vi "tankdata.vi"(7 "LabVIEW Web Service Request":refnum<class "Web Request.lvclass">) -> ()   [LabVIEW 2019]
uses:
  <vilib>/wsapi/Web Request.lvclass
  Type Defs/JSON_Channel.ctl
  Type Defs/JSON_Pump.ctl
panel:
  # "Use the Web Service Request input terminal to call the VIs on the Web Services palette. Do not remove it from the connector pane unless you don't need access to the palette."
  # "Each additional control wired to the connector pane will be available as an input in the URL. To include an indicator in terminal-mode output (the default setting), it must also be wired to the connector pane."
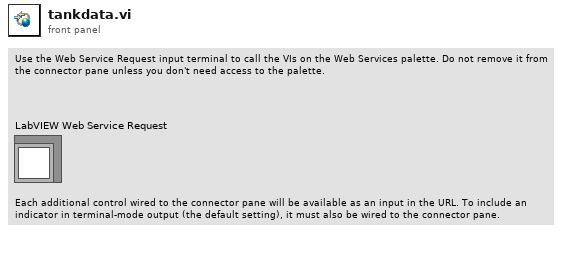
[diagram p1: front panel]
types:
  T1 = typedef "JSON_Tank.ctl" = cluster{"number":u16, "building":string, "room":string, "ipAddress":string, "profileName":string, "caNumber":string, "ctrlType":string, "mode":string, "channels":T2[], "pumps":T3[]}
  T2 = typedef "JSON_Channel.ctl" = cluster{"name":string, "tag":string, "data":string, "type":string, "unit":string}
  T3 = typedef "JSON_Pump.ctl" = cluster{"position":u8, "enabled":bool, "command":string, "channels":T2[], "elapsedTime":string}
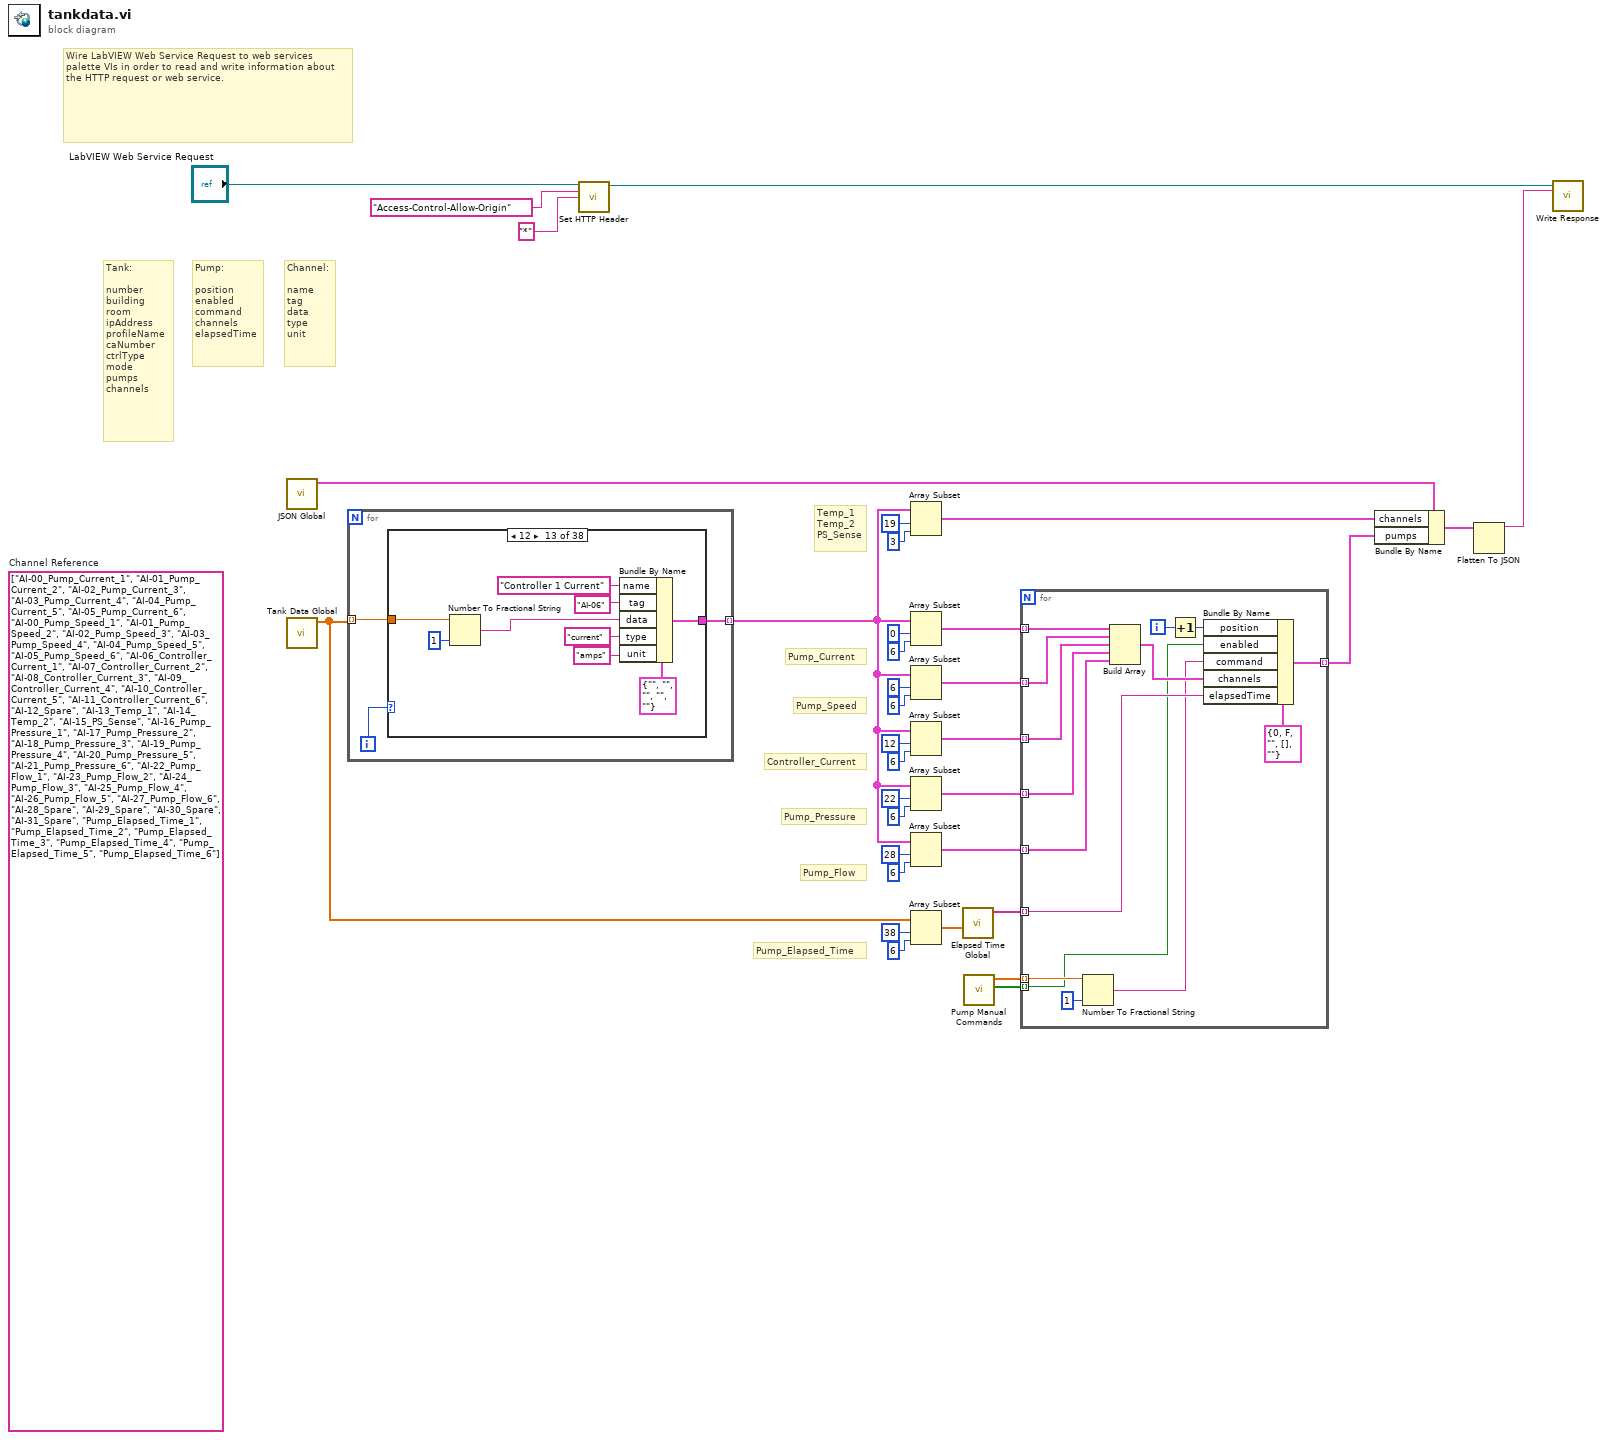
[diagram p0: block diagram]
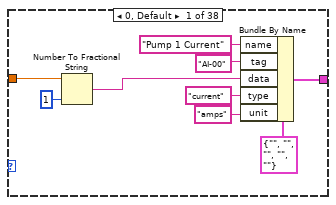
[diagram p2: hidden frame]
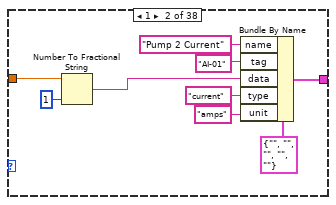
[diagram p3: hidden frame]
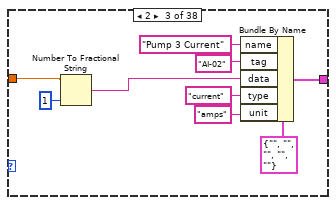
[diagram p4: hidden frame]
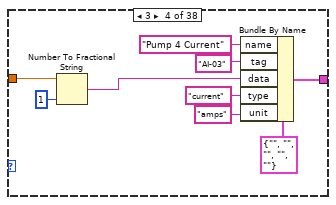
[diagram p5: hidden frame]
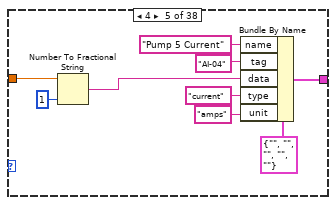
[diagram p6: hidden frame]
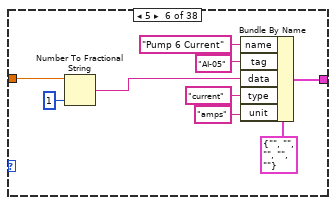
[diagram p7: hidden frame]
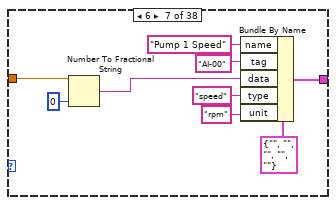
[diagram p8: hidden frame]
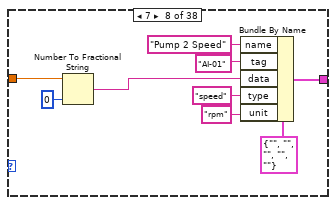
[diagram p9: hidden frame]
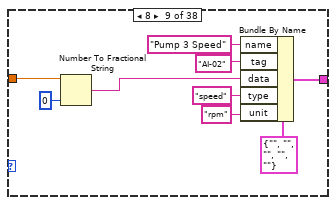
[diagram p10: hidden frame]
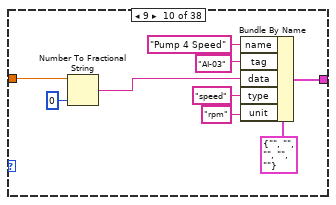
[diagram p11: hidden frame]
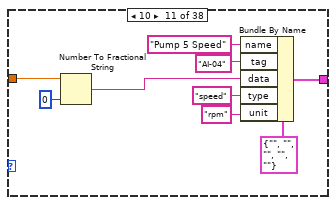
[diagram p12: hidden frame]
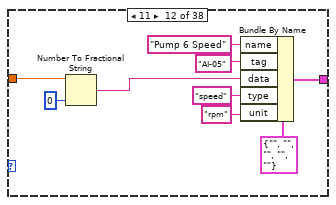
[diagram p13: hidden frame]
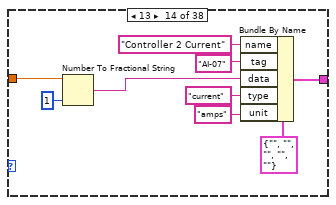
[diagram p14: hidden frame]
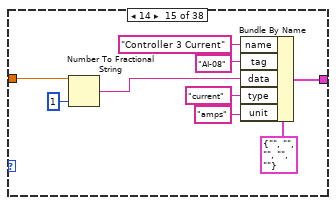
[diagram p15: hidden frame]
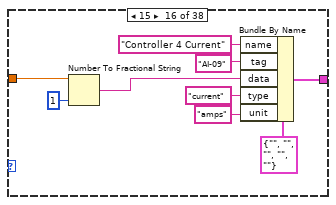
[diagram p16: hidden frame]
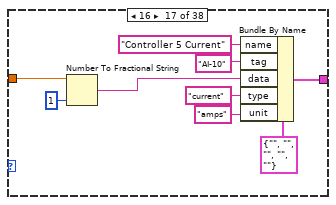
[diagram p17: hidden frame]
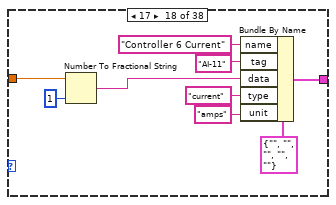
[diagram p18: hidden frame]
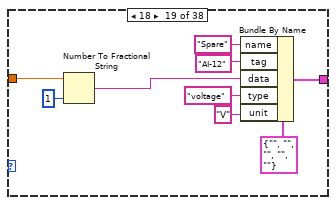
[diagram p19: hidden frame]
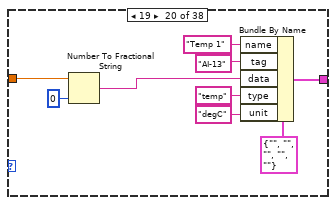
[diagram p20: hidden frame]
diagram:
  (unwired) string[] ["AI-00_Pump_Current_1", "AI-01_Pump_Current_2", "AI-02_Pump_Current_3", "AI-03_Pump_Current_4", "AI-04_Pump_Current_5", "AI-05_Pump_Current_6", "AI-00_Pump_Speed_1", "AI-01_Pump_Speed_2", "AI-02_Pump_Speed_3", "AI-03_Pump_Speed_4", "AI-04_Pump_Speed_5", "AI-05_Pump_Speed_6", "AI-06_Controller_Current_1", "AI-07_Controller_Current_2", "AI-08_Controller_Current_3", "AI-09_Controller_Current_4", "AI-10_Controller_Current_5", "AI-11_Controller_Current_6", "AI-12_Spare", "AI-13_Temp_1", "AI-14_Temp_2", "AI-15_PS_Sense", "AI-16_Pump_Pressure_1", "AI-17_Pump_Pressure_2", "AI-18_Pump_Pressure_3", "AI-19_Pump_Pressure_4", "AI-20_Pump_Pressure_5", "AI-21_Pump_Pressure_6", "AI-22_Pump_Flow_1", "AI-23_Pump_Flow_2", "AI-24_Pump_Flow_3", "AI-25_Pump_Flow_4", "AI-26_Pump_Flow_5", "AI-27_Pump_Flow_6", "AI-28_Spare", "AI-29_Spare", "AI-30_Spare", "AI-31_Spare", "Pump_Elapsed_Time_1", "Pump_Elapsed_Time_2", "Pump_Elapsed_Time_3", "Pump_Elapsed_Time_4", "Pump_Elapsed_Time_5", "Pump_Elapsed_Time_6"]  # Channel Reference
  # "Temp_1\nTemp_2\nPS_Sense"
  # "Pump_Elapsed_Time"
  # "Pump_Flow"
  # "Pump_Pressure"
  # "Controller_Current"
  # "Pump_Speed"
  # "Pump_Current"
  # "Tank:\n\nnumber\nbuilding\nroom\nipAddress\nprofileName\ncaNumber\nctrlType\nmode\npumps\nchannels"
  # "Channel:\n\nname\ntag\ndata\ntype\nunit"
  # "Pump:\n\nposition\nenabled\ncommand\nchannels\nelapsedTime"
  # "Wire LabVIEW Web Service Request to web services palette VIs in order to read and write information about the HTTP request or web service."
  n1 = call "JSON Global.vi"() -> ("JSON Out"=w12:T1)  [unwired: 11 in]
  n2 = call "Tank Data Global.vi"() -> ("Tank Data OUT"=w1:dbl[])  [unwired: 11 in]
  n3 = for {
    tunnel: w1 -> [w36] mode=indexing
    tunnel: [w35] -> w9 mode=indexing
    i -> [w37]
    n4 = case shown="12" w37 {
      tunnel: w36 -> [w39 w48 w57 w66 w75 w84 w93 w102 w111 w120 w129 w138 w147 w156 w165 w174 w183 w192 w201 w210 w219 w228 w237 w246 w255 w264 w273 w282 w291 w300 w309 w318 w327 w336 w345 w354 w363 w372]
      tunnel: [w45 w54 w63 w72 w81 w90 w99 w108 w117 w126 w135 w144 w153 w162 w171 w180 w189 w198 w207 w216 w225 w234 w243 w252 w261 w270 w279 w288 w297 w306 w315 w324 w333 w342 w351 w360 w369 w378] -> w35
      frame 0, Default {
        n5 = Number To Fractional String(number=w39, precision (6)=i16 1) -> (F-format string=w38:string)  [unwired: 2 in]
        n6 = Bundle By Name(cluster=T2 {"name"="", "tag"="", "data"="", "type"="", "unit"=""} ("Cluster"), "name"="Pump 1 Current", "tag"="AI-00" ("name"), "data"=w38, "type"="current", "unit"="amps") -> (w45:T2)
      }
      frame 1 {
        n7 = Number To Fractional String(number=w48, precision (6)=i16 1) -> (F-format string=w47:string)  [unwired: 2 in]
        n8 = Bundle By Name(cluster=T2 {"name"="", "tag"="", "data"="", "type"="", "unit"=""} ("Cluster"), "name"="Pump 2 Current", "tag"="AI-01" ("name"), "data"=w47, "type"="current", "unit"="amps") -> (w54:T2)
      }
      frame 2 {
        n9 = Number To Fractional String(number=w57, precision (6)=i16 1) -> (F-format string=w56:string)  [unwired: 2 in]
        n10 = Bundle By Name(cluster=T2 {"name"="", "tag"="", "data"="", "type"="", "unit"=""} ("Cluster"), "name"="Pump 3 Current", "tag"="AI-02" ("name"), "data"=w56, "type"="current", "unit"="amps") -> (w63:T2)
      }
      frame 3 {
        n11 = Number To Fractional String(number=w66, precision (6)=i16 1) -> (F-format string=w65:string)  [unwired: 2 in]
        n12 = Bundle By Name(cluster=T2 {"name"="", "tag"="", "data"="", "type"="", "unit"=""} ("Cluster"), "name"="Pump 4 Current", "tag"="AI-03" ("name"), "data"=w65, "type"="current", "unit"="amps") -> (w72:T2)
      }
      frame 4 {
        n13 = Number To Fractional String(number=w75, precision (6)=i16 1) -> (F-format string=w74:string)  [unwired: 2 in]
        n14 = Bundle By Name(cluster=T2 {"name"="", "tag"="", "data"="", "type"="", "unit"=""} ("Cluster"), "name"="Pump 5 Current", "tag"="AI-04" ("name"), "data"=w74, "type"="current", "unit"="amps") -> (w81:T2)
      }
      frame 5 {
        n15 = Number To Fractional String(number=w84, precision (6)=i16 1) -> (F-format string=w83:string)  [unwired: 2 in]
        n16 = Bundle By Name(cluster=T2 {"name"="", "tag"="", "data"="", "type"="", "unit"=""} ("Cluster"), "name"="Pump 6 Current", "tag"="AI-05" ("name"), "data"=w83, "type"="current", "unit"="amps") -> (w90:T2)
      }
      frame 6 {
        n17 = Number To Fractional String(number=w93, precision (6)=i16 0) -> (F-format string=w92:string)  [unwired: 2 in]
        n18 = Bundle By Name(cluster=T2 {"name"="", "tag"="", "data"="", "type"="", "unit"=""} ("Cluster"), "name"="Pump 1 Speed", "tag"="AI-00" ("name"), "data"=w92, "type"="speed", "unit"="rpm") -> (w99:T2)
      }
      frame 7 {
        n19 = Number To Fractional String(number=w102, precision (6)=i16 0) -> (F-format string=w101:string)  [unwired: 2 in]
        n20 = Bundle By Name(cluster=T2 {"name"="", "tag"="", "data"="", "type"="", "unit"=""} ("Cluster"), "name"="Pump 2 Speed", "tag"="AI-01" ("name"), "data"=w101, "type"="speed", "unit"="rpm") -> (w108:T2)
      }
      frame 8 {
        n21 = Number To Fractional String(number=w111, precision (6)=i16 0) -> (F-format string=w110:string)  [unwired: 2 in]
        n22 = Bundle By Name(cluster=T2 {"name"="", "tag"="", "data"="", "type"="", "unit"=""} ("Cluster"), "name"="Pump 3 Speed", "tag"="AI-02" ("name"), "data"=w110, "type"="speed", "unit"="rpm") -> (w117:T2)
      }
      frame 9 {
        n23 = Number To Fractional String(number=w120, precision (6)=i16 0) -> (F-format string=w119:string)  [unwired: 2 in]
        n24 = Bundle By Name(cluster=T2 {"name"="", "tag"="", "data"="", "type"="", "unit"=""} ("Cluster"), "name"="Pump 4 Speed", "tag"="AI-03" ("name"), "data"=w119, "type"="speed", "unit"="rpm") -> (w126:T2)
      }
      frame 10 {
        n25 = Number To Fractional String(number=w129, precision (6)=i16 0) -> (F-format string=w128:string)  [unwired: 2 in]
        n26 = Bundle By Name(cluster=T2 {"name"="", "tag"="", "data"="", "type"="", "unit"=""} ("Cluster"), "name"="Pump 5 Speed", "tag"="AI-04" ("name"), "data"=w128, "type"="speed", "unit"="rpm") -> (w135:T2)
      }
      frame 11 {
        n27 = Number To Fractional String(number=w138, precision (6)=i16 0) -> (F-format string=w137:string)  [unwired: 2 in]
        n28 = Bundle By Name(cluster=T2 {"name"="", "tag"="", "data"="", "type"="", "unit"=""} ("Cluster"), "name"="Pump 6 Speed", "tag"="AI-05" ("name"), "data"=w137, "type"="speed", "unit"="rpm") -> (w144:T2)
      }
      frame 12 {
        n29 = Number To Fractional String(number=w147, precision (6)=i16 1) -> (F-format string=w146:string)  [unwired: 2 in]
        n30 = Bundle By Name(cluster=T2 {"name"="", "tag"="", "data"="", "type"="", "unit"=""} ("Cluster"), "name"="Controller 1 Current", "tag"="AI-06" ("name"), "data"=w146, "type"="current", "unit"="amps") -> (w153:T2)
      }
      frame 13 {
        n31 = Number To Fractional String(number=w156, precision (6)=i16 1) -> (F-format string=w155:string)  [unwired: 2 in]
        n32 = Bundle By Name(cluster=T2 {"name"="", "tag"="", "data"="", "type"="", "unit"=""} ("Cluster"), "name"="Controller 2 Current", "tag"="AI-07" ("name"), "data"=w155, "type"="current", "unit"="amps") -> (w162:T2)
      }
      frame 14 {
        n33 = Number To Fractional String(number=w165, precision (6)=i16 1) -> (F-format string=w164:string)  [unwired: 2 in]
        n34 = Bundle By Name(cluster=T2 {"name"="", "tag"="", "data"="", "type"="", "unit"=""} ("Cluster"), "name"="Controller 3 Current", "tag"="AI-08" ("name"), "data"=w164, "type"="current", "unit"="amps") -> (w171:T2)
      }
      frame 15 {
        n35 = Number To Fractional String(number=w174, precision (6)=i16 1) -> (F-format string=w173:string)  [unwired: 2 in]
        n36 = Bundle By Name(cluster=T2 {"name"="", "tag"="", "data"="", "type"="", "unit"=""} ("Cluster"), "name"="Controller 4 Current", "tag"="AI-09" ("name"), "data"=w173, "type"="current", "unit"="amps") -> (w180:T2)
      }
      frame 16 {
        n37 = Number To Fractional String(number=w183, precision (6)=i16 1) -> (F-format string=w182:string)  [unwired: 2 in]
        n38 = Bundle By Name(cluster=T2 {"name"="", "tag"="", "data"="", "type"="", "unit"=""} ("Cluster"), "name"="Controller 5 Current", "tag"="AI-10" ("name"), "data"=w182, "type"="current", "unit"="amps") -> (w189:T2)
      }
      frame 17 {
        n39 = Number To Fractional String(number=w192, precision (6)=i16 1) -> (F-format string=w191:string)  [unwired: 2 in]
        n40 = Bundle By Name(cluster=T2 {"name"="", "tag"="", "data"="", "type"="", "unit"=""} ("Cluster"), "name"="Controller 6 Current", "tag"="AI-11" ("name"), "data"=w191, "type"="current", "unit"="amps") -> (w198:T2)
      }
      frame 18 {
        n41 = Number To Fractional String(number=w201, precision (6)=i16 1) -> (F-format string=w200:string)  [unwired: 2 in]
        n42 = Bundle By Name(cluster=T2 {"name"="", "tag"="", "data"="", "type"="", "unit"=""} ("Cluster"), "name"="Spare", "tag"="AI-12" ("name"), "data"=w200, "type"="voltage", "unit"="V") -> (w207:T2)
      }
      frame 19 {
        n43 = Number To Fractional String(number=w210, precision (6)=i16 0) -> (F-format string=w209:string)  [unwired: 2 in]
        n44 = Bundle By Name(cluster=T2 {"name"="", "tag"="", "data"="", "type"="", "unit"=""} ("Cluster"), "name"="Temp 1", "tag"="AI-13" ("name"), "data"=w209, "type"="temp", "unit"="degC") -> (w216:T2)
      }
      frame 20 {
        n45 = Number To Fractional String(number=w219, precision (6)=i16 0) -> (F-format string=w218:string)  [unwired: 2 in]
        n46 = Bundle By Name(cluster=T2 {"name"="", "tag"="", "data"="", "type"="", "unit"=""} ("Cluster"), "name"="Temp 2", "tag"="AI-14" ("name"), "data"=w218, "type"="temp", "unit"="degC") -> (w225:T2)
      }
      frame 21 {
        n47 = Number To Fractional String(number=w228, precision (6)=i16 1) -> (F-format string=w227:string)  [unwired: 2 in]
        n48 = Bundle By Name(cluster=T2 {"name"="", "tag"="", "data"="", "type"="", "unit"=""} ("Cluster"), "name"="PS Sense", "tag"="AI-15" ("name"), "data"=w227, "type"="voltage", "unit"="V") -> (w234:T2)
      }
      frame 22 {
        n49 = Number To Fractional String(number=w237, precision (6)=i16 0) -> (F-format string=w236:string)  [unwired: 2 in]
        n50 = Bundle By Name(cluster=T2 {"name"="", "tag"="", "data"="", "type"="", "unit"=""} ("Cluster"), "name"="Pump 1 Pressure", "tag"="AI-16" ("name"), "data"=w236, "type"="pressure", "unit"="kPa") -> (w243:T2)
      }
      frame 23 {
        n51 = Number To Fractional String(number=w246, precision (6)=i16 0) -> (F-format string=w245:string)  [unwired: 2 in]
        n52 = Bundle By Name(cluster=T2 {"name"="", "tag"="", "data"="", "type"="", "unit"=""} ("Cluster"), "name"="Pump 2 Pressure", "tag"="AI-17" ("name"), "data"=w245, "type"="pressure", "unit"="kPa") -> (w252:T2)
      }
      frame 24 {
        n53 = Number To Fractional String(number=w255, precision (6)=i16 0) -> (F-format string=w254:string)  [unwired: 2 in]
        n54 = Bundle By Name(cluster=T2 {"name"="", "tag"="", "data"="", "type"="", "unit"=""} ("Cluster"), "name"="Pump 3 Pressure", "tag"="AI-18" ("name"), "data"=w254, "type"="pressure", "unit"="kPa") -> (w261:T2)
      }
      frame 25 {
        n55 = Number To Fractional String(number=w264, precision (6)=i16 0) -> (F-format string=w263:string)  [unwired: 2 in]
        n56 = Bundle By Name(cluster=T2 {"name"="", "tag"="", "data"="", "type"="", "unit"=""} ("Cluster"), "name"="Pump 4 Pressure", "tag"="AI-19" ("name"), "data"=w263, "type"="pressure", "unit"="kPa") -> (w270:T2)
      }
      frame 26 {
        n57 = Number To Fractional String(number=w273, precision (6)=i16 0) -> (F-format string=w272:string)  [unwired: 2 in]
        n58 = Bundle By Name(cluster=T2 {"name"="", "tag"="", "data"="", "type"="", "unit"=""} ("Cluster"), "name"="Pump 5 Pressure", "tag"="AI-20" ("name"), "data"=w272, "type"="pressure", "unit"="kPa") -> (w279:T2)
      }
      frame 27 {
        n59 = Number To Fractional String(number=w282, precision (6)=i16 0) -> (F-format string=w281:string)  [unwired: 2 in]
        n60 = Bundle By Name(cluster=T2 {"name"="", "tag"="", "data"="", "type"="", "unit"=""} ("Cluster"), "name"="Pump 6 Pressure", "tag"="AI-21" ("name"), "data"=w281, "type"="pressure", "unit"="kPa") -> (w288:T2)
      }
      frame 28 {
        n61 = Number To Fractional String(number=w291, precision (6)=i16 0) -> (F-format string=w290:string)  [unwired: 2 in]
        n62 = Bundle By Name(cluster=T2 {"name"="", "tag"="", "data"="", "type"="", "unit"=""} ("Cluster"), "name"="Pump 1 Flow", "tag"="AI-22" ("name"), "data"=w290, "type"="flow", "unit"="lph") -> (w297:T2)
      }
      frame 29 {
        n63 = Number To Fractional String(number=w300, precision (6)=i16 0) -> (F-format string=w299:string)  [unwired: 2 in]
        n64 = Bundle By Name(cluster=T2 {"name"="", "tag"="", "data"="", "type"="", "unit"=""} ("Cluster"), "name"="Pump 2 Flow", "tag"="AI-23" ("name"), "data"=w299, "type"="flow", "unit"="lph") -> (w306:T2)
      }
      frame 30 {
        n65 = Number To Fractional String(number=w309, precision (6)=i16 0) -> (F-format string=w308:string)  [unwired: 2 in]
        n66 = Bundle By Name(cluster=T2 {"name"="", "tag"="", "data"="", "type"="", "unit"=""} ("Cluster"), "name"="Pump 3 Flow", "tag"="AI-24" ("name"), "data"=w308, "type"="flow", "unit"="lph") -> (w315:T2)
      }
      frame 31 {
        n67 = Number To Fractional String(number=w318, precision (6)=i16 0) -> (F-format string=w317:string)  [unwired: 2 in]
        n68 = Bundle By Name(cluster=T2 {"name"="", "tag"="", "data"="", "type"="", "unit"=""} ("Cluster"), "name"="Pump 4 Flow", "tag"="AI-25" ("name"), "data"=w317, "type"="flow", "unit"="lph") -> (w324:T2)
      }
      frame 32 {
        n69 = Number To Fractional String(number=w327, precision (6)=i16 0) -> (F-format string=w326:string)  [unwired: 2 in]
        n70 = Bundle By Name(cluster=T2 {"name"="", "tag"="", "data"="", "type"="", "unit"=""} ("Cluster"), "name"="Pump 5 Flow", "tag"="AI-26" ("name"), "data"=w326, "type"="flow", "unit"="lph") -> (w333:T2)
      }
      frame 33 {
        n71 = Number To Fractional String(number=w336, precision (6)=i16 0) -> (F-format string=w335:string)  [unwired: 2 in]
        n72 = Bundle By Name(cluster=T2 {"name"="", "tag"="", "data"="", "type"="", "unit"=""} ("Cluster"), "name"="Pump 6 Flow", "tag"="AI-27" ("name"), "data"=w335, "type"="flow", "unit"="lph") -> (w342:T2)
      }
      frame 34 {
        n73 = Number To Fractional String(number=w345, precision (6)=i16 1) -> (F-format string=w344:string)  [unwired: 2 in]
        n74 = Bundle By Name(cluster=T2 {"name"="", "tag"="", "data"="", "type"="", "unit"=""} ("Cluster"), "name"="Spare", "tag"="AI-28" ("name"), "data"=w344, "type"="voltage", "unit"="V") -> (w351:T2)
      }
      frame 35 {
        n75 = Number To Fractional String(number=w354, precision (6)=i16 1) -> (F-format string=w353:string)  [unwired: 2 in]
        n76 = Bundle By Name(cluster=T2 {"name"="", "tag"="", "data"="", "type"="", "unit"=""} ("Cluster"), "name"="Spare", "tag"="AI-29" ("name"), "data"=w353, "type"="voltage", "unit"="V") -> (w360:T2)
      }
      frame 36 {
        n77 = Number To Fractional String(number=w363, precision (6)=i16 1) -> (F-format string=w362:string)  [unwired: 2 in]
        n78 = Bundle By Name(cluster=T2 {"name"="", "tag"="", "data"="", "type"="", "unit"=""} ("Cluster"), "name"="Spare", "tag"="AI-30" ("name"), "data"=w362, "type"="voltage", "unit"="V") -> (w369:T2)
      }
      frame 37 {
        n79 = Number To Fractional String(number=w372, precision (6)=i16 1) -> (F-format string=w371:string)  [unwired: 2 in]
        n80 = Bundle By Name(cluster=T2 {"name"="", "tag"="", "data"="", "type"="", "unit"=""} ("Cluster"), "name"="Spare", "tag"="AI-31" ("name"), "data"=w371, "type"="voltage", "unit"="V") -> (w378:T2)
      }
    }
  }
  n81 = call <vilib>:"Set HTTP Header.vi"("LabVIEW Web Service Request"="LabVIEW Web Service Request", "header"="Access-Control-Allow-Origin" ("header value"), "header value"="*" ("header")) -> ("LabVIEW Web Service Request out"=w33:refnum<class "Web Request.lvclass">)  [unwired: 11 in, 1 out]
  n82 = Array Subset(array=w9, index=19, length=3 ("index")) -> (w8:T2[])
  n83 = Array Subset(array=w9, index=0, length=6 ("index")) -> (w18:T2[])
  n84 = Array Subset(array=w9, index=6, length=6 ("index")) -> (w17:T2[])
  n85 = Array Subset(array=w9, index=12, length=6 ("index")) -> (w16:T2[])
  n86 = Array Subset(array=w9, index=22, length=6 ("index")) -> (w15:T2[])
  n87 = Array Subset(array=w9, index=28, length=6 ("index")) -> (w14:T2[])
  n88 = Array Subset(array=w1, index=38, length=6 ("index")) -> (w13:dbl[])
  n89 = call "Elapsed Time Global.vi"("Ticks IN"=w13) -> ("Elapsed Times"=w4:string[])  [unwired: 10 in]
  n90 = call "Pump Manual Commands.vi"() -> ("Pumps Enabled OUT"=w2:bool[], "Manual CMDs OUT"=w3:dbl[])  [unwired: 10 in]
  n91 = for {
    tunnel: w18 -> [w394] mode=indexing
    tunnel: w17 -> [w393] mode=indexing
    tunnel: w16 -> [w392] mode=indexing
    tunnel: w15 -> [w391] mode=indexing
    tunnel: w14 -> [w390] mode=indexing
    tunnel: w4 -> [w386] mode=indexing
    tunnel: [w385] -> w7 mode=indexing
    tunnel: w3 -> [w382] mode=indexing
    tunnel: w2 -> [w380] mode=indexing
    i -> [w388]
    n92 = Number To Fractional String(number=w382, precision (6)=i16 1) -> (F-format string=w381:string)  [unwired: 2 in]
    n93 = Build Array(w394, w393, w392, w391, w390) -> (w387:T2[])
    n94 = Increment(x=w388) -> (x+1=w384:i32)
    n95 = Bundle By Name(cluster=T3 {"position"=0, "enabled"=FALSE, "command"="", "channels"=[], "elapsedTime"=""}, "position"=w384, "enabled"=w380, "command"=w381, "channels"=w387, "elapsedTime"=w386) -> (w385:T3)
  }
  n96 = Bundle By Name(cluster=w12, "channels"=w8, "pumps"=w7) -> (w6:T1)
  n97 = Flatten To JSON(anything=w6) -> (JSON string=w5:string)  [unwired: 2 in, 1 out]
  n98 = call <vilib>:"Write Response.vi"("LabVIEW Web Service Request"=w33, "response string"=w5) -> ()  [unwired: 12 in, 2 out]
